vi "_keysight_status.vi"(0 "error in":errorcluster, 3 "Connection":T2={"Type"=1, "VISA"="TCPIP0::192.168.0.8::inst0::INSTR", "GPIB"="10"} {"Type" items=["VISA", "GPIB"]}) -> (1 "error out":errorcluster, 4 "Keysight settings":T1 {"Frequency 1 (Hz)" format="%#_6p"; "Frequency 2 (Hz)" format="%#_6p"})   [LabVIEW 2013]
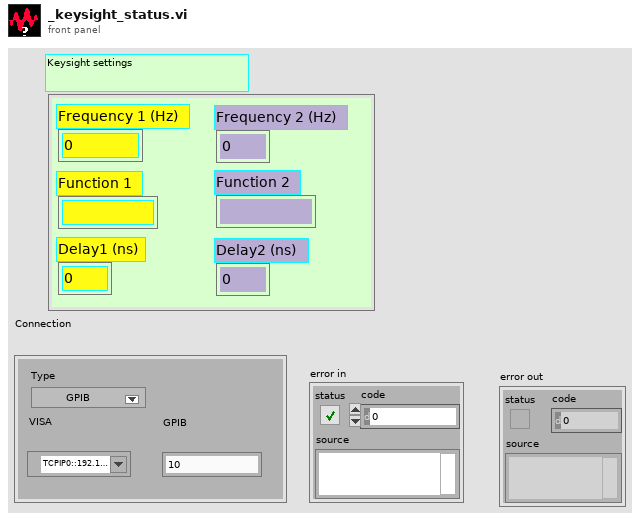
[diagram p1: front panel]
types:
  T1 = cluster{"Frequency 2 (Hz)":dbl, "Function 2":string, "Delay2 (ns) ":dbl, "Frequency 1 (Hz)":dbl, "Function 1":string, "Delay1 (ns)":dbl}
  T2 = cluster{"Type":u16, "VISA":refnum<visa-resource-name>, "GPIB":string}
  T3 = cluster{dbl, "Raw output":string, dbl, dbl, "Raw output":string, dbl}
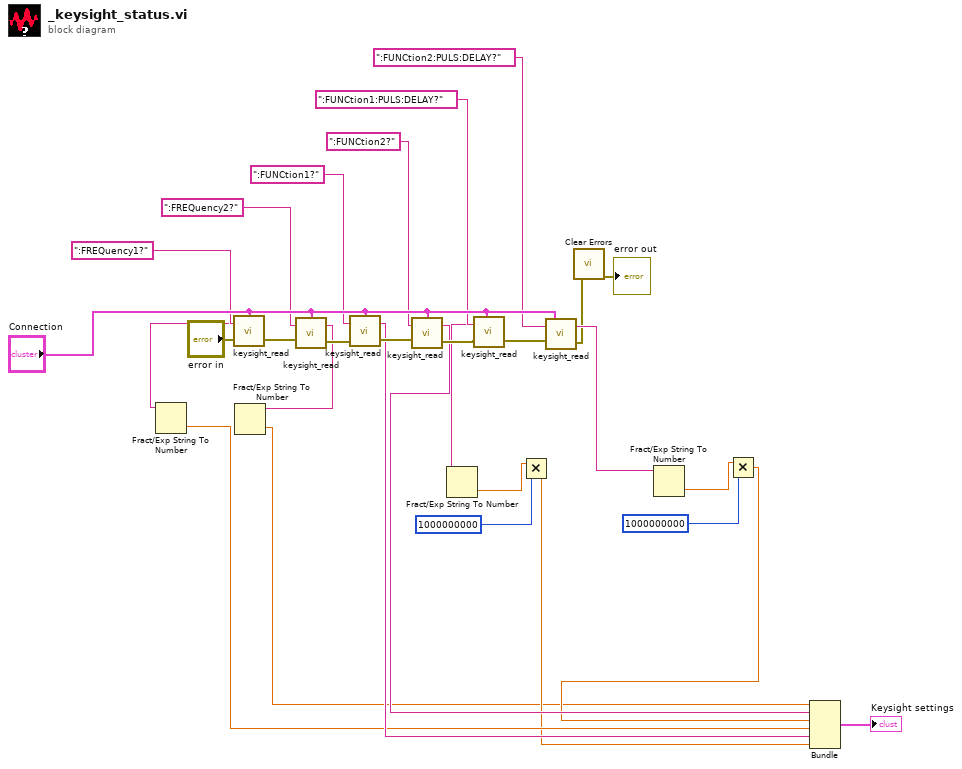
[diagram p0: block diagram]
diagram:
  n1 = call "keysight_read.vi"("error in"="error in", "command"=":FREQuency1?", "Connection"="Connection") -> ("error out"=w30:errorcluster, "Raw output"=w18:string)
  n2 = Fract/Exp String To Number(string=w18) -> (number=w5:dbl)  [unwired: 3 in, 1 out]
  n3 = call "keysight_read.vi"("error in"=w30, "command"=":FREQuency2?", "Connection"="Connection") -> ("error out"=w29:errorcluster, "Raw output"=w17:string)
  n4 = Fract/Exp String To Number(string=w17) -> (number=w2:dbl)  [unwired: 3 in, 1 out]
  n5 = call "keysight_read.vi"("error in"=w29, "command"=":FUNCtion1?", "Connection"="Connection") -> ("error out"=w28:errorcluster, "Raw output"=w6:string)
  n6 = call "keysight_read.vi"("error in"=w28, "command"=":FUNCtion2?", "Connection"="Connection") -> ("error out"=w27:errorcluster, "Raw output"=w7:string)
  n7 = call "keysight_read.vi"("error in"=w27, "command"=":FUNCtion1:PULS:DELAY?", "Connection"="Connection") -> ("error out"=w26:errorcluster, "Raw output"=w8:string)
  n8 = Fract/Exp String To Number(string=w8) -> (number=w15:dbl)  [unwired: 3 in, 1 out]
  n9 = Multiply(x=w15, y=1000000000) -> (x*y=w4:dbl)
  n10 = call "keysight_read.vi"("error in"=w26, "command"=":FUNCtion2:PULS:DELAY?", "Connection"="Connection") -> ("error out"=w10:errorcluster, "Raw output"=w12:string)
  n11 = call <vilib>:"Clear Errors.vi"("error in (no error)"=w10) -> ("error out"=→"error out":errorcluster)  [unwired: 6 in]
  n12 = Fract/Exp String To Number(string=w12) -> (number=w13:dbl)  [unwired: 3 in, 1 out]
  n13 = Multiply(x=w13, y=1000000000) -> (x*y=w3:dbl)
  n14 = Bundle(w2, "Raw output"=w7, w3, w5, "Raw output"=w6, w4) -> (→"Keysight settings":T3)  [unwired: 1 in]
